vi "Stop HD Recorder.vi"(8 "error in (no error)":errorcluster, 9 "Frames":i32, 10 "Wait for completion":bool, 11 "Orca-Flash 4.0 V2 in":refnum<class "Orca-Flash 4.0 V2.lvclass">) -> (0 "error out":errorcluster, 3 "Orca-Flash 4.0 V2 out":refnum<class "Orca-Flash 4.0 V2.lvclass">)   [LabVIEW 2015, in "Orca-Flash 4.0 V2.lvlib" / "Orca-Flash 4.0 V2.lvclass"]
uses:
  Orca-Flash 4.0 V2.lvclass
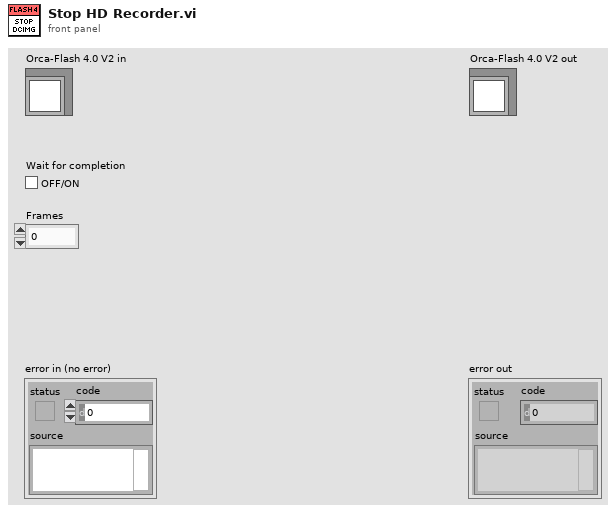
[diagram p1: front panel]
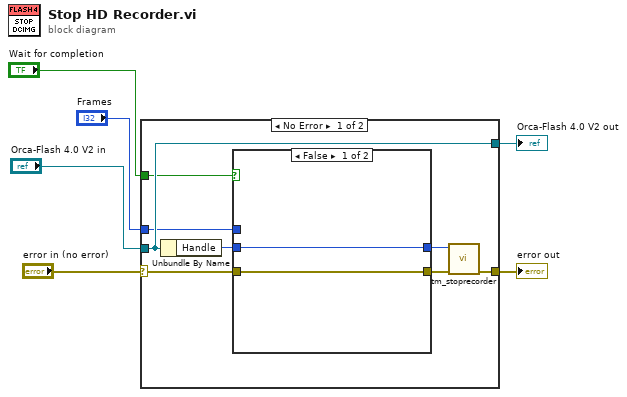
[diagram p0: block diagram]
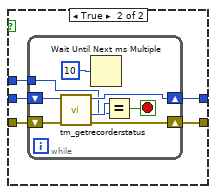
[diagram p2: hidden frame]
diagram:
  n1 = case shown="No Error" "error in (no error)" {
    selector: "error in (no error)" -> [w10 w31]
    tunnel: [w8 w31] -> w5
    tunnel: [w14 w30] -> w3
    tunnel: "Orca-Flash 4.0 V2 in" -> [w14 w30]
    tunnel: "Frames" -> [w12 _]
    tunnel: "Wait for completion" -> [w7 _]
    frame No Error {
      n2 = Unbundle By Name(w14) -> ("Handle"=w13:u32)
      n3 = case shown="False" w7 {
        tunnel: w13 -> [w16 w21]
        tunnel: w12 -> [_ w20]
        tunnel: [w16 w19] -> w11
        tunnel: w10 -> [w15 w18]
        tunnel: [w15 w17] -> w9
        frame False {
        }
        frame True {
          n4 = while {
            shift-right: [w28] -> w19
            shift-left: w21 -> [w29]
            tunnel: w20 -> [w25]
            shift-right: [w22] -> w17
            shift-left: w18 -> [w23]
            stop <- w24 stop-if-true
            n5 = call <userlib>:"tm_getrecorderstatus.vi"("error in (no error)"=w23, "Handle"=w29) -> ("error out"=w22:errorcluster, "Count"=w26:i32, "Handle"=w28:u32)  [unwired: 6 in, 1 out]
            n6 = Wait Until Next ms Multiple(millisecond multiple=u32 10) -> ()  [unwired: 1 out]
            n7 = Equal?(x=w26, y=w25) -> (x = y?=w24:bool)
          }
        }
      }
      n8 = call <userlib>:"tm_stoprecorder.vi"("error in (no error)"=w9, "Handle in"=w11) -> ("error out"=w8:errorcluster)  [unwired: 8 in, 1 out]
    }
    frame Error {
    }
  }
  "error out" <- w5
  "Orca-Flash 4.0 V2 out" <- w3
